vi "UMLEditor EvaluationDialog.vi"(5 "error in (no error)":errorcluster) -> (15 "PassWord":string="HTTP/1.0 200 OK\r\nDate: Mon, 28 Apr 2003 08:45:03 GMT\r\nServer: Apache/1.3.20 (Unix) ApacheJServ/1.1.2 PHP/4.2.3 FrontPage/5.0.2.2510 Rewrit/1.1a\r\nContent-Type: text/html\r\nX-Cache: MISS from 217.75.96.62\r\nX-Cache-Lookup: MISS from 217.75.96.62:3128\r\nConnection: close\r\n\r\n<p>Hello, micke!</p>\n<p>holmstrom</p>\n", 19 "error out":errorcluster)   [LabVIEW 2016]
panel:
  in  "Cancel Button":bool
  in  "OK Button":bool
  in  "e-mail":string
  in  "Name":string
  out "Text1":string="HTTP/1.0 200 OK\r\nDate: Mon, 28 Apr 2003 08:45:03 GMT\r\nServer: Apache/1.3.20 (Unix) ApacheJServ/1.1.2 PHP/4.2.3 FrontPage/5.0.2.2510 Rewrit/1.1a\r\nContent-Type: text/html\r\nX-Cache: MISS from 217.75.96.62\r\nX-Cache-Lookup: MISS from 217.75.96.62:3128\r\nConnection: close\r\n\r\n<p>Hello, micke!</p>\n<p>holmstrom</p>\n"
  # "Welcome to this evaluation version of this UML-editor\n\nBefore you can start, you have to registrate this version:\nEnter the information below and then press send.\n(You have to be connected to the internet)"
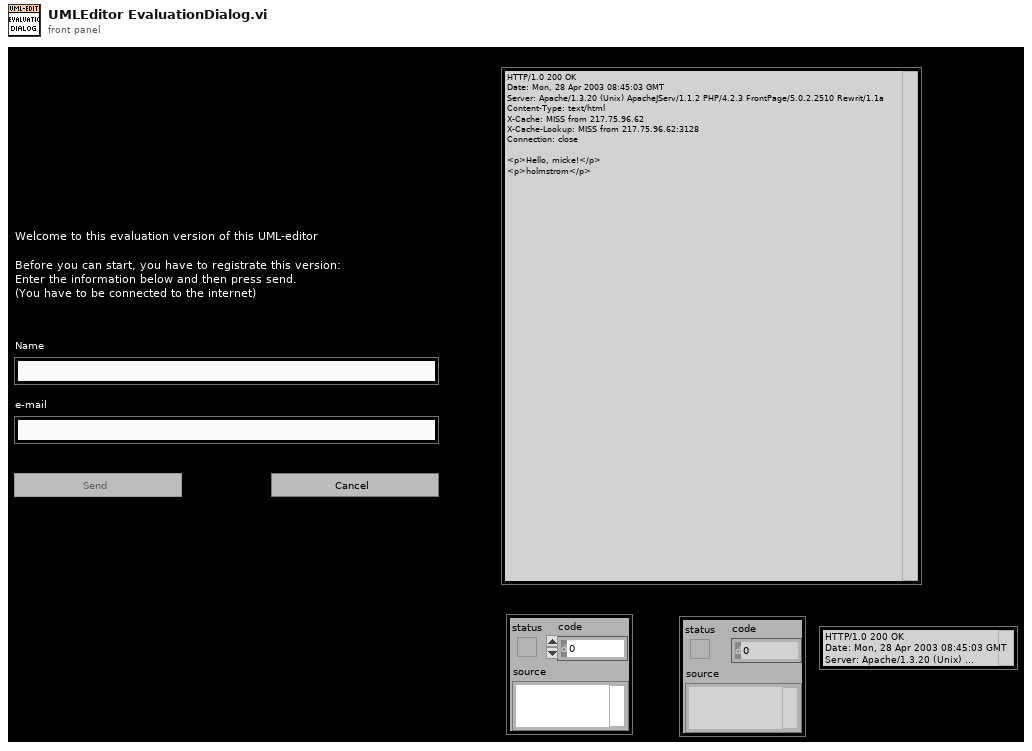
[diagram p1: front panel]
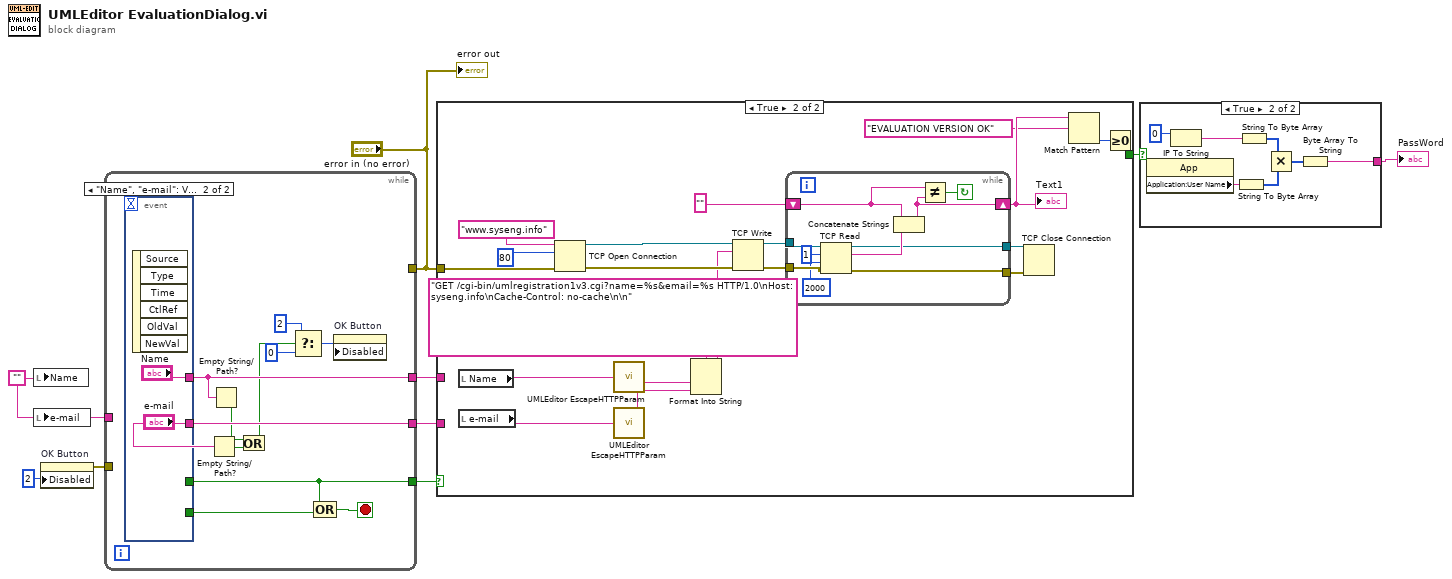
[diagram p0: block diagram]
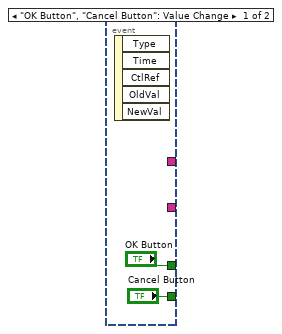
[diagram p2: hidden frame]
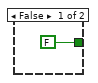
[diagram p3: hidden frame]
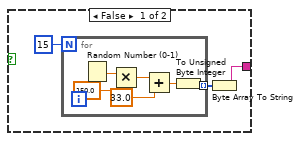
[diagram p4: hidden frame]
diagram:
  w2 = ""
  n1 = local write "Name"(w2) -> ()
  n2 = local write "e-mail"(w2) -> ()
  n3 = property on="OK Button" class="Bool"("Disabled"=u8 2) -> (error out=w3:errorcluster)  [unwired: 2 in, 1 out]
  n4 = while {
    tunnel: "error in (no error)" -> [_]
    tunnel: [w20] -> w7
    tunnel: [w19] -> w6
    tunnel: [w10] -> w5
    tunnel: w3 -> [_]
    tunnel: w2 -> [_]
    stop <- w16 stop-if-true
    n5 = event shown="[1] \"Name\", \"e-mail\": Value Change" {
      selector: _ -> [_ _]
      dyn-events: _ -> [_ _]
      timeout: _ -> [_ _]
      tunnel: [_ "Name"] -> w20
      tunnel: [_ "e-mail"] -> w19
      tunnel: ["OK Button" _] -> w10
      tunnel: ["Cancel Button" _] -> w12
      event "OK Button", "Cancel Button": Value Change {
        n6 = event-data() -> ()  [unwired: 6 out]
      }
      event "Name", "e-mail": Value Change {
        n7 = event-data() -> ()  [unwired: 7 out]
      }
    }
    n8 = Empty String/Path?(string/path=w19) -> (empty?=w18:bool)
    n9 = Empty String/Path?(string/path=w20) -> (empty?=w17:bool)
    n10 = Or(x=w17, y=w18) -> (x .or. y?=w11:bool)
    n11 = Select(t=u8 2 ("Disabled"), s=w11, f=u8 0) -> (s? t:f=w14:u8)
    n12 = Compound Arithmetic op=OR(w10, w12) -> (w16:bool)
    n13 = property on="OK Button" class="Bool"("Disabled"=w14) -> ()  [unwired: 2 in, 2 out]
  }
  n14 = case shown="True" w5 {
    tunnel: "error in (no error)" -> [_ w32]
    tunnel: [FALSE w28] -> w9
    tunnel: w7 -> [_ _]
    tunnel: w6 -> [_ _]
    frame False {
    }
    frame True {
      n15 = local read "Name"() -> (w26:string)
      n16 = local read "e-mail"() -> (w27:string)
      n17 = TCP Open Connection(address="www.syseng.info", remote port or service name=u16 80 ("remote port"), error in (no error)=w32) -> (connection ID=w38:refnum<k5>, error out=w37:errorcluster)  [unwired: 2 out]
      n18 = call <resource>:"UMLEditor EscapeHTTPParam.vi"("string"=w26) -> ("url-encoded string"=w34:string)
      n19 = call <resource>:"UMLEditor EscapeHTTPParam.vi"("string"=w27) -> ("url-encoded string"=w33:string)
      n20 = Format Into String(format string="GET /cgi-bin/umlregistration1v3.cgi?name=%s&email=%s HTTP/1.0\nHost: syseng.info\nCache-Control: no-cache\n\n" ("Text sent"), w34, w33) -> (resulting string=w35:string)  [unwired: 2 in, 1 out]
      n21 = TCP Write(connection ID=w38, data in=w35, error in (no error)=w37) -> (connection ID out=w44:refnum<k5>, error out=w43:errorcluster)  [unwired: 2 out]
      n22 = while {
        tunnel: [w46] -> w41
        tunnel: [w48] -> w42
        tunnel: w43 -> [w49]
        shift-left: "" ("address") -> [w52]
        shift-right: [w51] -> w31
        tunnel: w44 -> [w55]
        stop <- w50 continue-if-true
        n23 = TCP Read(connection ID=w55, bytes to read=1, error in (no error)=w49, 9:2000 ("timeout ms (25000)")) -> (connection ID out=w48:refnum<k5>, data out=w53:string, error out=w46:errorcluster)  [unwired: 1 out]
        n24 = Concatenate Strings(w52, w53) -> (w51:string)
        n25 = Not Equal?(x=w52, y=w51) -> (x != y?=w50:bool)
      }
      "Text1" <- w31
      n26 = TCP Close Connection(connection ID=w42, error in (no error)=w41) -> ()  [unwired: 3 out]
      n27 = Match Pattern(string=w31, regular expression="EVALUATION VERSION OK") -> (offset past match=w29:i32)  [unwired: 4 out]
      n28 = Greater Or Equal To 0?(x=w29) -> (x >= 0?=w28:bool)
    }
  }
  n29 = case shown="True" w9 {
    tunnel: [w56 w65] -> w8
    frame False {
      n30 = for {
        N: 15 -> [_]
        tunnel: [w59] -> w57 mode=indexing
        n31 = Random Number (0-1)() -> (number: 0 to 1=w64:dbl)
        n32 = Multiply(x=w64, y=150.0) -> (x*y=w62:dbl)
        n33 = Add(x=w62, y=33.0) -> (x+y=w60:dbl)
        n34 = To Unsigned Byte Integer(number=w60) -> (unsigned 8bit integer=w59:u8)
      }
      n35 = Byte Array To String(unsigned byte array=w57) -> (string=w56:string)
    }
    frame True {
      n36 = property class="App"() -> ("Application:User Name"=w70:string)  [unwired: 2 in, 2 out]
      n37 = IP To String(2:u32 0 ("net address")) -> (0:w69:string)  [unwired: 1 out]
      n38 = String To Byte Array(string=w70) -> (unsigned byte array=w67:u8[])
      n39 = String To Byte Array(string=w69) -> (unsigned byte array=w68:u8[])
      n40 = Multiply(x=w68, y=w67) -> (x*y=w66:u8[])
      n41 = Byte Array To String(unsigned byte array=w66) -> (string=w65:string)
    }
  }
  "PassWord" <- w8
  "error out" <- "error in (no error)"
